vi "Set Measurement Name Voltage-QPOET.vi"(8 "error in (no error)":errorcluster, 10 "Meas Name In":string, 11 "Message in":refnum<class "String Database.lvclass">) -> (0 "error out":errorcluster, 2 "Meas Name Out":string, 3 "Message out":refnum<class "String Database.lvclass">)   [LabVIEW 2016, in "QPA Measurement.lvlib" / "QPA Measurement.lvclass"]
uses:
  QPA Measurement.lvclass
  Plugins/String Database.lvlibp/String Database.lvclass
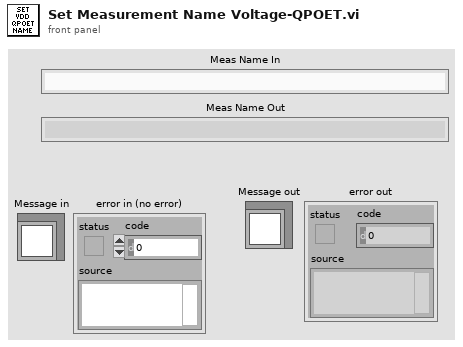
[diagram p1: front panel]
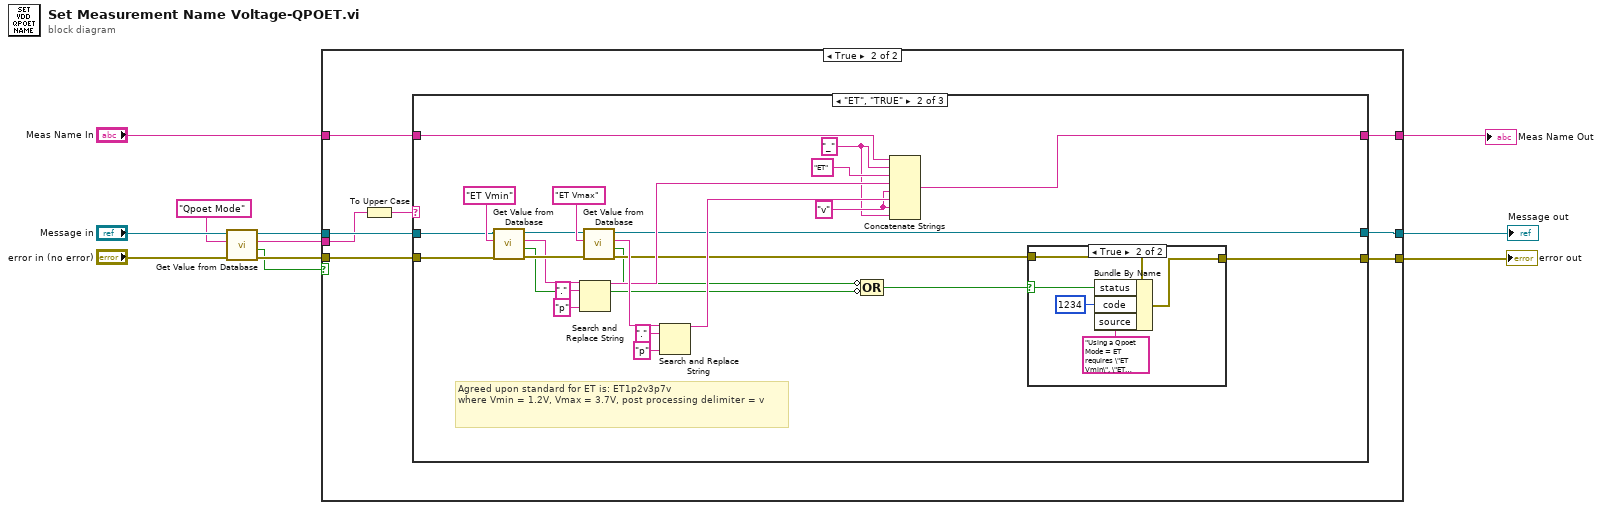
[diagram p0: block diagram]
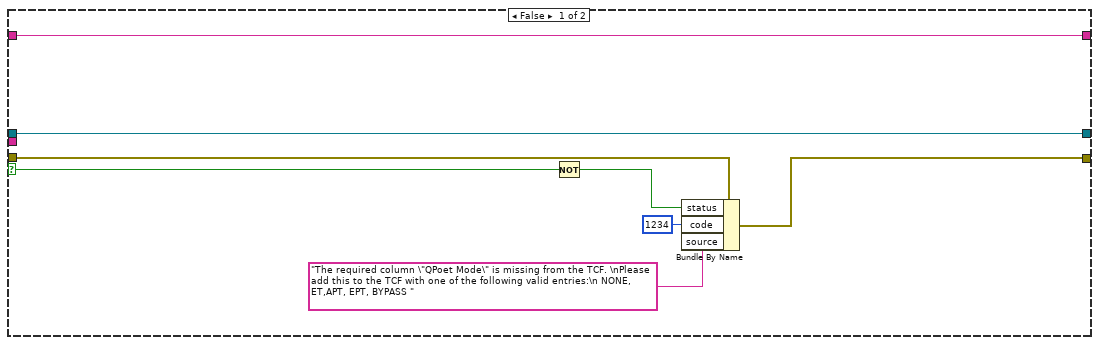
[diagram p2: hidden frame]
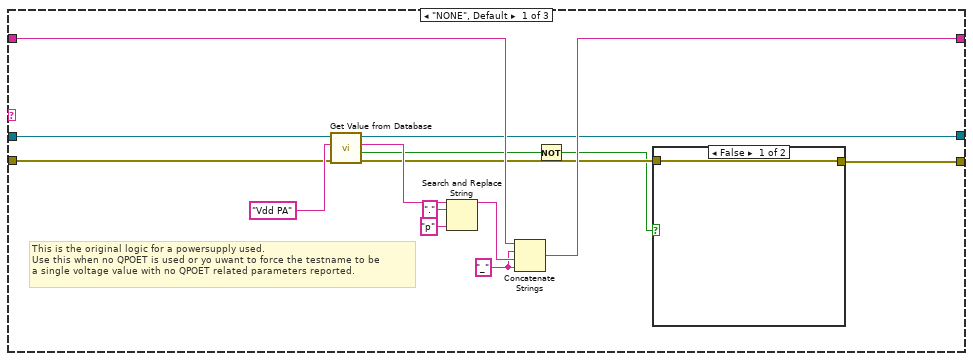
[diagram p3: hidden frame]
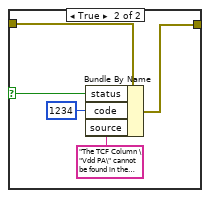
[diagram p4: hidden frame]
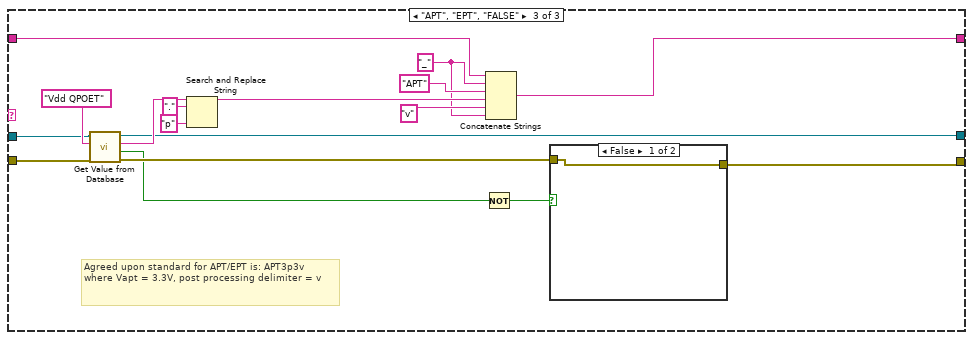
[diagram p6: hidden frame]
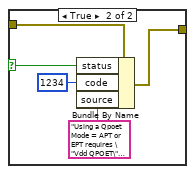
[diagram p7: hidden frame]
diagram:
  n1 = call "Get Value from Database.vi"("error in (no error)"="error in (no error)", "Entry Name"="Qpoet Mode", "Message in"="Message in") -> ("error out"=w8:errorcluster, "Entry Found"=w1:bool, "Entry Value"=w6:string, "Message out"=w7:refnum<class "String Database.lvclass">)  [unwired: 5 in]
  n2 = case shown="True" w1 {
    selector: w1 -> [w15 _]
    tunnel: w8 -> [w17 w27]
    tunnel: w7 -> [w19 w26]
    tunnel: w6 -> [_ w25]
    tunnel: "Meas Name In" -> [w12 w24]
    tunnel: [w12 w23] -> w4
    tunnel: [w16 w21] -> w3
    tunnel: [w19 w20] -> w2
    frame False {
      n3 = Not(x=w15) -> (.not. x?=w14:bool)
      n4 = Bundle By Name(cluster=w17, "status"=w14, "code"=1234, "source"="The required column \"QPoet Mode\" is missing from the TCF. \nPlease add this to the TCF with one of the following valid entries:\n NONE, ET,APT, EPT, BYPASS " ("string")) -> (w16:errorcluster)
    }
    frame True {
      n5 = To Upper Case(1:w25) -> (0:w22:string)
      n6 = case shown="\"ET\", \"TRUE\"" w22 {
        tunnel: w27 -> [w33 w72 w95]
        tunnel: w26 -> [w36 w71 w94]
        tunnel: w24 -> [w35 w57 w87]
        tunnel: [w34 w56 w86] -> w23
        tunnel: [w31 w54 w85] -> w21
        tunnel: [w32 w51 w82] -> w20
        frame "NONE", Default {
          w37 = "_" ("string")
          # "This is the original logic for a powersupply used.\nUse this when no QPOET is used or yo uwant to force the testname to be\na single voltage value with no QPOET related parameters reported."
          n7 = call "Get Value from Database.vi"("error in (no error)"=w33, "Entry Name"="Vdd PA", "Message in"=w36) -> ("error out"=w30:errorcluster, "Entry Found"=w29:bool, "Entry Value"=w41:string, "Message out"=w32:refnum<class "String Database.lvclass">)  [unwired: 5 in]
          n8 = Search and Replace String(input string=w41, search string=".", replace string="p" ("replace string (\"\")")) -> (result string=w38:string)  [unwired: 5 in, 3 out]
          n9 = Concatenate Strings(w35, w37, w38, w37) -> (w34:string)
          n10 = Not(x=w29) -> (.not. x?=w28:bool)
          n11 = case shown="False" w28 {
            selector: w28 -> [_ w44]
            tunnel: [w43 w46] -> w31
            tunnel: w30 -> [w43 w45]
            frame False {
            }
            frame True {
              n12 = Bundle By Name(cluster=w45, "status"=w44, "code"=1234, "source"="The TCF Column \"Vdd PA\" cannot be found in the TCF.  This defines the Vdd of the PA when not using QPOET (Qpoet Mode = NONE)." ("string")) -> (w46:errorcluster)
            }
          }
        }
        frame "ET", "TRUE" {
          w58 = "v" ("string")
          w50 = "_" ("string")
          # "Agreed upon standard for ET is: ET1p2v3p7v \nwhere Vmin = 1.2V, Vmax = 3.7V, post processing delimiter = v"
          n13 = call "Get Value from Database.vi"("error in (no error)"=w72, "Entry Name"="ET Vmin", "Message in"=w71) -> ("error out"=w69:errorcluster, "Entry Found"=w53:bool, "Entry Value"=w65:string, "Message out"=w68:refnum<class "String Database.lvclass">)  [unwired: 5 in]
          n14 = Search and Replace String(input string=w65, search string=".", replace string="p" ("replace string (\"\")")) -> (result string=w60:string)  [unwired: 5 in, 3 out]
          n15 = call "Get Value from Database.vi"("error in (no error)"=w69, "Entry Name"="ET Vmax", "Message in"=w68) -> ("error out"=w55:errorcluster, "Entry Found"=w52:bool, "Entry Value"=w62:string, "Message out"=w51:refnum<class "String Database.lvclass">)  [unwired: 5 in]
          n16 = Search and Replace String(input string=w62, search string=".", replace string="p" ("replace string (\"\")")) -> (result string=w59:string)  [unwired: 5 in, 3 out]
          n17 = Compound Arithmetic op=OR(invert w52, invert w53) -> (w49:bool)
          n18 = Concatenate Strings(w57, w50, "ET" ("string"), w60, w58, w59, w58, w50) -> (w56:string)
          n19 = case shown="True" w49 {
            selector: w49 -> [_ w75]
            tunnel: w55 -> [w74 w79]
            tunnel: [w74 w78] -> w54
            frame False {
            }
            frame True {
              n20 = Bundle By Name(cluster=w79, "status"=w75, "code"=1234, "source"="Using a Qpoet Mode = ET requires \"ET Vmin\", \"ET Vmax\" columns  to be present in the TCF. \nPlease add these columns to your TCF or change the Qpoet mode." ("string")) -> (w78:errorcluster)
            }
          }
        }
        frame "APT", "EPT", "FALSE" {
          w81 = "_" ("string")
          # "Agreed upon standard for APT/EPT is: APT3p3v \nwhere Vapt = 3.3V, post processing delimiter = v"
          n21 = call "Get Value from Database.vi"("error in (no error)"=w95, "Entry Name"="Vdd QPOET", "Message in"=w94) -> ("error out"=w84:errorcluster, "Entry Found"=w83:bool, "Entry Value"=w91:string, "Message out"=w82:refnum<class "String Database.lvclass">)  [unwired: 5 in]
          n22 = Search and Replace String(input string=w91, search string=".", replace string="p" ("replace string (\"\")")) -> (result string=w89:string)  [unwired: 5 in, 3 out]
          n23 = Not(x=w83) -> (.not. x?=w80:bool)
          n24 = Concatenate Strings(w87, w81, "APT" ("string"), w89, "v" ("string"), w81) -> (w86:string)
          n25 = case shown="False" w80 {
            selector: w80 -> [_ w98]
            tunnel: [w97 w100] -> w85
            tunnel: w84 -> [w97 w99]
            frame False {
            }
            frame True {
              n26 = Bundle By Name(cluster=w99, "status"=w98, "code"=1234, "source"="Using a Qpoet Mode = APT or EPT requires \"Vdd QPOET\" column  to be present in the TCF. \nPlease add this column to your TCF or change the Qpoet mode." ("string")) -> (w100:errorcluster)
            }
          }
        }
      }
    }
  }
  "Message out" <- w2
  "error out" <- w3
  "Meas Name Out" <- w4
